vi "Create DSFPlugin.vi"(8 "error in (no error)":errorcluster, 9 "DSFPlugin info":T1, 10 "id":string, 11 "DSFPlugin in":refnum<class "DSFPlugin.lvclass">) -> (0 "error out":errorcluster, 3 "DSFPlugin out":refnum<class "DSFPlugin.lvclass">)   [LabVIEW 2017, in "DSFPlugin.lvclass"]
uses:
  DSFPlugin.lvclass
  DSFTiming/DSFTiming.lvclass
  DSFPlugin.lvclass/DSFPlugin.ctl
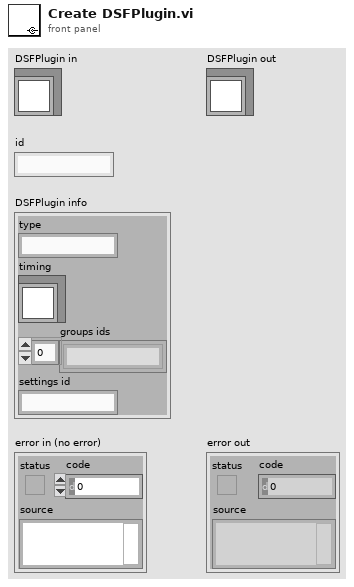
[diagram p1: front panel]
types:
  T1 = cluster{"type":string, "timing":refnum<class "DSFTiming.lvclass">, "groups ids":string[], "settings id":string}
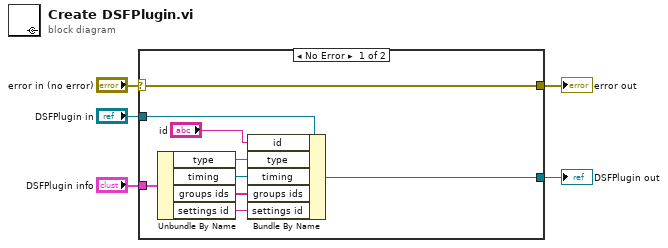
[diagram p0: block diagram]
diagram:
  n1 = case shown="No Error" "error in (no error)" {
    selector: "error in (no error)" -> [w14 w16]
    tunnel: [w14 w16] -> w4
    tunnel: [w12 w15] -> w2
    tunnel: "DSFPlugin in" -> [w13 w15]
    tunnel: "DSFPlugin info" -> [w10 _]
    frame No Error {
      n2 = Unbundle By Name(w10) -> ("type"=w9:string, "timing"=w8:refnum<class "DSFTiming.lvclass">, "groups ids"=w7:string[], "settings id"=w6:string)
      n3 = Bundle By Name(cluster=w13, "id"="id", "type"=w9, "timing"=w8, "groups ids"=w7, "settings id"=w6) -> (w12:refnum<class "DSFPlugin.lvclass">)
    }
    frame Error {
    }
  }
  "error out" <- w4
  "DSFPlugin out" <- w2
